vi "meTEC_Send & Read Serial Message.vi"(7 "VISA resource name":refnum<visa-resource-name>, 8 "error in (no error)":errorcluster, 11 "Serial Message":string) -> (0 "error out":errorcluster, 3 "Serial Message_Read":string)   [LabVIEW 2019]
panel:
  out "Return Count [Bytes]":u32
  # "--- Outputs ---"
  # "--- Inputs ---"
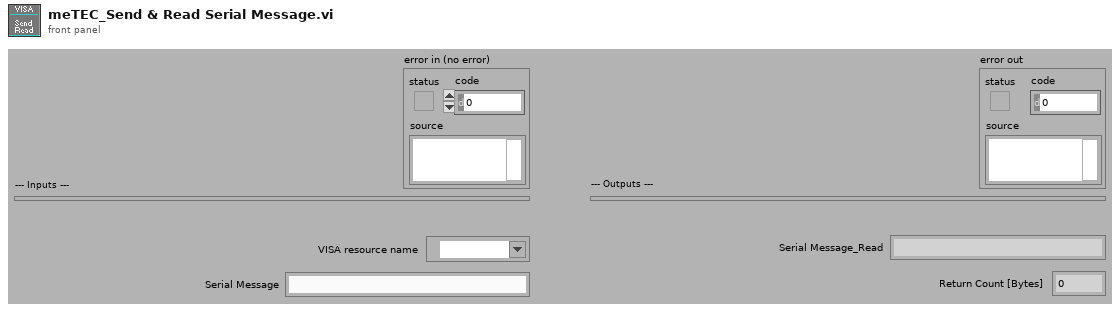
[diagram p1: front panel]
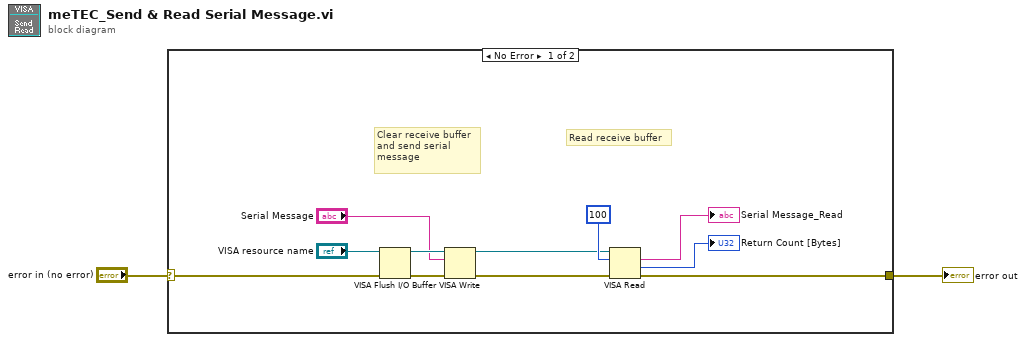
[diagram p0: block diagram]
diagram:
  n1 = case shown="No Error" "error in (no error)" {
    selector: "error in (no error)" -> [w12 w14]
    tunnel: [w8 w14] -> w2
    frame No Error {
      # "Read receive buffer"
      # "Clear receive buffer\nand send serial\nmessage"
      n2 = VISA Flush I/O Buffer(VISA resource name="VISA resource name", error in (no error)=w12) -> (VISA resource name out=w13:refnum<visa-resource-name>, error out=w11:errorcluster)  [unwired: 1 in]
      n3 = VISA Write(VISA resource name=w13, write buffer="Serial Message", error in (no error)=w11) -> (VISA resource name out=w4:refnum<visa-resource-name>, error out=w3:errorcluster)  [unwired: 1 out]
      n4 = VISA Read(VISA resource name=w4, byte count=u32 100, error in (no error)=w3) -> (read buffer=→"Serial Message_Read":string, return count=→"Return Count [Bytes]":u32, error out=w8:errorcluster)  [unwired: 1 out]
    }
    frame Error {
    }
  }
  "error out" <- w2
